vi "CAN State to String.vi"(11 "CAN comm in":T1 {"fault code" format="%08x"; "last error" items=["None", "Stuff", "Form", "Ack", "Bit1", "Bit0", "CRC"]; "communication state" items=["Error Active", "Error Passive", "Bus Off", "Init"]}) -> (3 "string out":string)   [LabVIEW 2025, in "CAN-LIN Raw Bus Capture.lvclass"]
uses:
  CAN-LIN Raw Bus Capture.lvclass
  <vilib>/xnet/xnet.llb/XNET CAN Comm.ctl
  <vilib>/xnet/xnet.llb/XNET CAN Comm State.ctl
  <vilib>/xnet/xnet.llb/XNET CAN Last Err.ctl
  CAN-LIN Raw Bus Capture.lvclass/CAN-LIN Raw Bus Capture.ctl
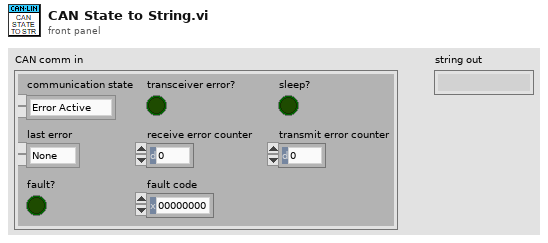
[diagram p1: front panel]
types:
  T1 = typedef "XNET CAN Comm.ctl" = cluster{"fault code":i32, "fault?":bool, "communication state":T2, "last error":T3, "receive error counter":u8, "transmit error counter":u8, "transceiver error?":bool, "sleep?":bool}
  T2 = typedef "XNET CAN Comm State.ctl" = u8
  T3 = typedef "XNET CAN Last Err.ctl" = u8
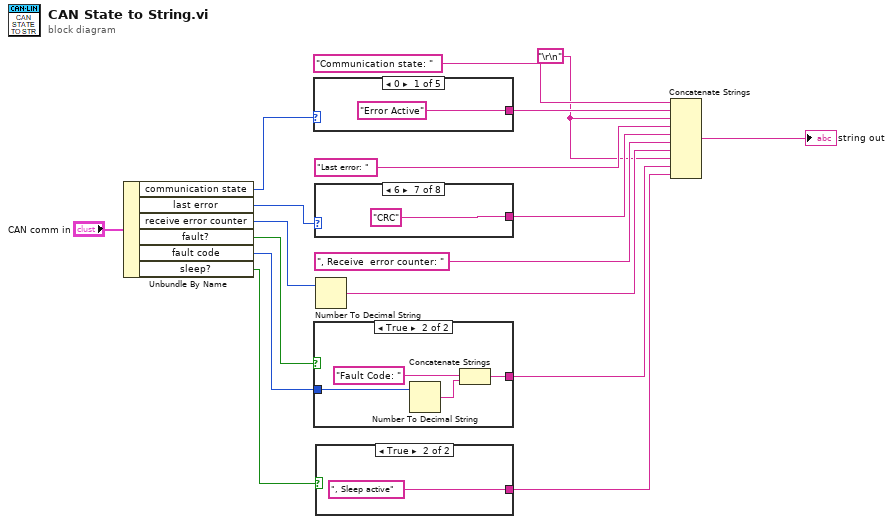
[diagram p0: block diagram]
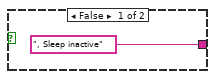
[diagram p2: hidden frame]
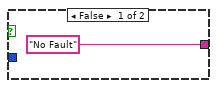
[diagram p3: hidden frame]
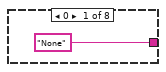
[diagram p4: hidden frame]
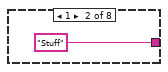
[diagram p5: hidden frame]
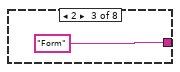
[diagram p6: hidden frame]
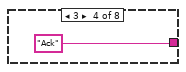
[diagram p7: hidden frame]
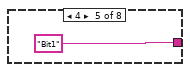
[diagram p8: hidden frame]
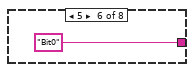
[diagram p9: hidden frame]
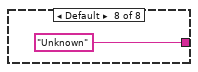
[diagram p10: hidden frame]
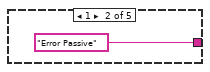
[diagram p11: hidden frame]
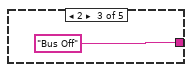
[diagram p12: hidden frame]
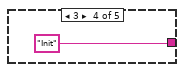
[diagram p13: hidden frame]
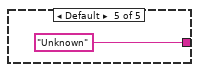
[diagram p14: hidden frame]
diagram:
  w4 = "\r\n"
  n1 = Unbundle By Name("CAN comm in") -> ("communication state"=w15:T2, "last error"=w9:T3, "receive error counter"=w8:u8, "fault?"=w7:bool, "fault code"=w6:i32, "sleep?"=w3:bool)
  n2 = case shown="0" w15 {
    tunnel: ["Error Active" ("string") "Error Passive" ("string") "Bus Off" ("string") "Init" ("string") "Unknown" ("string")] -> w14
    frame 0 {
    }
    frame 1 {
    }
    frame 2 {
    }
    frame 3 {
    }
    frame Default {
    }
  }
  n3 = case shown="True" w7 {
    tunnel: w6 -> [_ w27]
    tunnel: ["No Fault" ("string") w24] -> w5
    frame False {
    }
    frame True {
      n4 = Number To Decimal String(number=w27) -> (decimal integer string=w25:string)  [unwired: 1 in]
      n5 = Concatenate Strings("Fault Code: " ("string"), w25) -> (w24:string)
    }
  }
  n6 = case shown="6" w9 {
    tunnel: ["None" ("string") "Stuff" ("string") "Form" ("string") "Ack" ("string") "Bit1" ("string") "Bit0" ("string") "CRC" ("string") "Unknown" ("string")] -> w12
    frame 0 {
    }
    frame 1 {
    }
    frame 2 {
    }
    frame 3 {
    }
    frame 4 {
    }
    frame 5 {
    }
    frame 6 {
    }
    frame Default {
    }
  }
  n7 = Number To Decimal String(number=w8) -> (decimal integer string=w10:string)  [unwired: 1 in]
  n8 = case shown="True" w3 {
    tunnel: [", Sleep inactive" ("string") ", Sleep active" ("string")] -> w2
    frame False {
    }
    frame True {
    }
  }
  n9 = Concatenate Strings("Communication state: " ("string"), w14, w4, "Last error: " ("string"), w12, ", Receive  error counter: " ("string"), w10, w4, w5, w2) -> (→"string out":string)
